vi "práctica3.vi"() -> ()   [LabVIEW 2018]
uses:
  <vilib>/addons/Wavelet Analysis/continuous wavelet transform.llb/WA Continuous Wavelet Transform (Waveform).vi
  <vilib>/addons/_Advanced Signal Processing/NI_AdvSigProcWA.lvlib
panel:
  out "CWT Coefficients Cumulation":dbl[](graph)
  in  "stop":bool
  out "Waveform Graph 2":waveform(dbl)(graph)
  out "Waveform Graph":dynamicdata(graph)
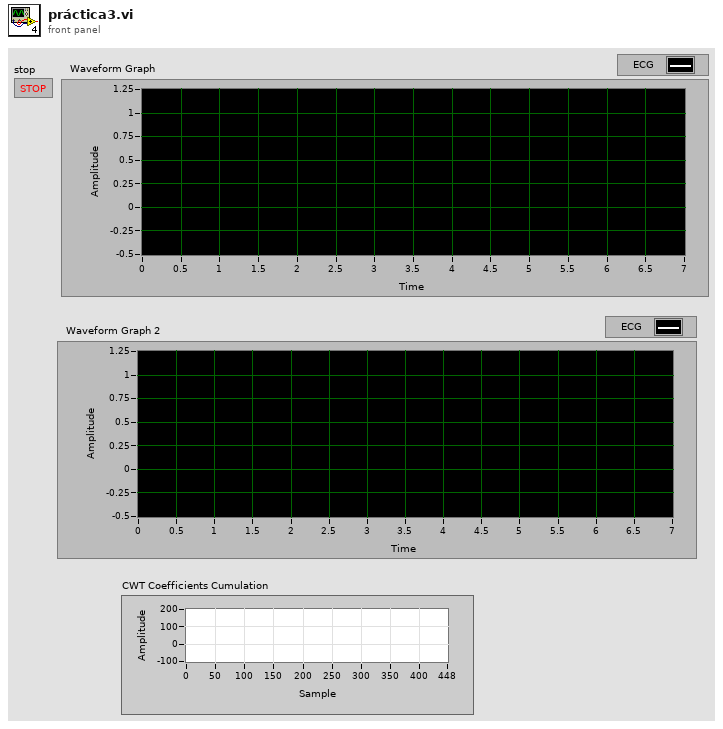
[diagram p1: front panel]
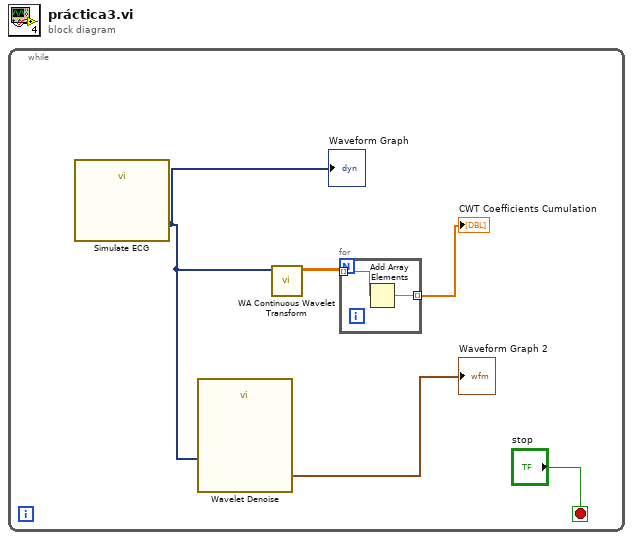
[diagram p0: block diagram]
diagram:
  n1 = while {
    stop <- "stop" stop-if-true
    n2 = call "Simulate ECG"() -> ("ECG"=w4:dynamicdata)  [unwired: 10 in, 1 out]
    "Waveform Graph" <- w4
    n3 = call "Wavelet Denoise"("Signal"=w4) -> ("Denoised Signal"=→"Waveform Graph 2":waveform(dbl))  [unwired: 9 in, 1 out]
    n4 = call-poly <vilib>:"WA Continuous Wavelet Transform.vi"("signal"=w4) -> ("CWT coef"=w2:dbl[][])  [unwired: 8 in, 2 out]
    n5 = for {
      tunnel: w2 -> [w7] mode=indexing
      tunnel: [w6] -> w1 mode=indexing
      n6 = Add Array Elements(numeric array=w7) -> (sum=w6:dbl)
    }
    "CWT Coefficients Cumulation" <- w1
  }
